vi "SetParam.vi"(8 "error in (no error)":errorcluster caption="entrée d'erreur (pas d'erreur)", 10 "ParameterGrid":T1, 11 "ParameterGrid.lvclass":refnum<class "ParameterGrid.lvclass">) -> (0 "error out":errorcluster caption="sortie d'erreur", 3 "ParameterGrid.lvclass":refnum<class "ParameterGrid.lvclass">)   [LabVIEW 2020, in "ParameterGrid.lvclass"]
doc: "Set Parameters"
uses:
  ParameterGrid.lvclass
  ParameterGrid.lvclass/ParameterGrid.ctl
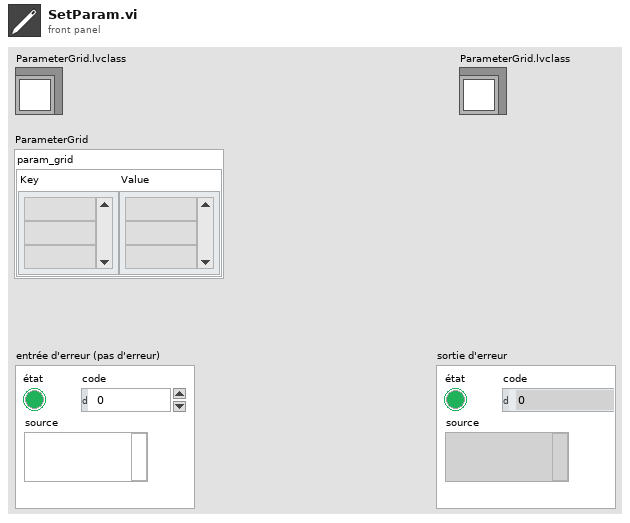
[diagram p1: front panel]
types:
  T1 = cluster{"param_grid":cluster{"Key":string[], "Value":string[]}}
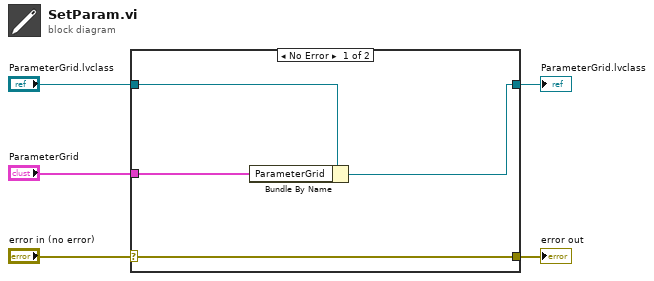
[diagram p0: block diagram]
diagram:
  n1 = case shown="No Error" "error in (no error)" {
    selector: "error in (no error)" -> [w9 w10]
    tunnel: [w9 w10] -> w4
    tunnel: [w7 w11] -> w2
    tunnel: "ParameterGrid.lvclass" -> [w8 w11]
    tunnel: "ParameterGrid" -> [w6 _]
    frame No Error {
      n2 = Bundle By Name(cluster=w8, "ParameterGrid"=w6) -> (w7:refnum<class "ParameterGrid.lvclass">)
    }
    frame Error {
    }
  }
  "error out" <- w4
  "ParameterGrid.lvclass" <- w2
